vi "FirstInFirstOut.vi"(11 "Input":dbl) -> (3 "Output":dbl[](array[numeric]))   [LabVIEW 2017]
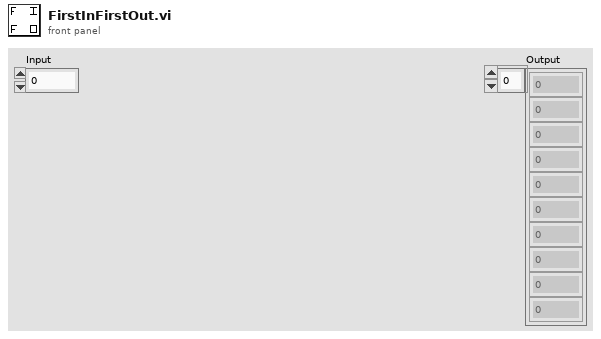
[diagram p1: front panel]
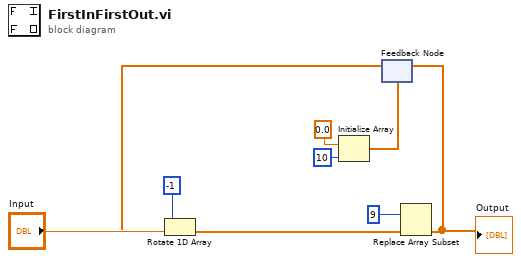
[diagram p0: block diagram]
diagram:
  n1 = Initialize Array(0.0, 10 ("dimension size")) -> (w3:dbl[])
  n2 = feedback #1(w3) -> (w2:dbl[])
  n3 = Rotate 1D Array(1:w2, 2:-1 ("n")) -> (0:w5:dbl[])
  n4 = Replace Array Subset(array=w5, new element="Input", index=9) -> (w1:dbl[])
  "Output" <- w1
  n5 = feedback-in #1(w1) -> ()
